vi "CapsLockEvent.vi"(0 "Input String":string, 7 "stop":bool) -> ()   [LabVIEW 2020]
doc: "This VI is done to implement keyboard , panel based filtering event to change the common functionality\nand configure it as per our requirement"
panel:
  # "Enter the input string to test the caps lock event \nand the front panel close is mapped to close and \ntermination of the program"
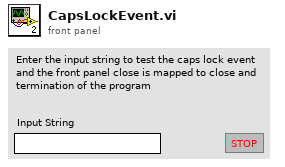
[diagram p1: front panel]
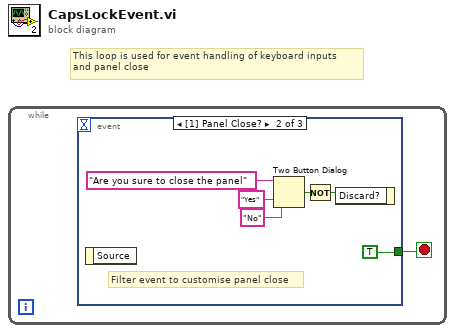
[diagram p0: block diagram]
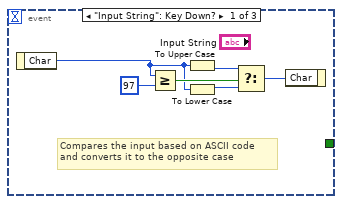
[diagram p2: hidden frame]
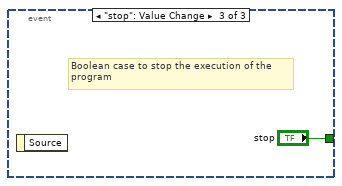
[diagram p3: hidden frame]
diagram:
  # "This loop is used for event handling of keyboard inputs\nand panel close"
  n1 = while {
    stop <- w1 stop-if-true
    n2 = event shown="[1] Panel Close?" {
      selector: _ -> [_ _ _]
      dyn-events: _ -> [_ _ _]
      timeout: _ -> [_ _ _]
      tunnel: [_ TRUE ("y") "stop"] -> w1
      event "Input String": Key Down? {
        # "Compares the input based on ASCII code\nand converts it to the opposite case"
        n3 = event-data() -> ("Char"=w5:i16)  [unwired: 1 in]
        n4 = Greater Or Equal?(x=w5, y=i16 97) -> (x >= y?=w7:bool)
        n5 = To Upper Case(1:w5) -> (0:w3:i16)
        n6 = To Lower Case(string=w5) -> (all lower case string=w4:i16)
        n7 = Select(t=w3, s=w7, f=w4) -> (s? t:f=w2:i16)
        n8 = event-data("Char"=w2) -> ()  [unwired: 1 in, 1 out]
      }
      event Panel Close? {
        # "Filter event to customise panel close"
        n9 = event-data() -> ()  [unwired: 1 in, 1 out]
        n10 = Two Button Dialog(message="Are you sure to close the panel", 1:"No" ("F button name (\"Cancel\")"), 2:"Yes" ("T button name (\"OK\")")) -> (T button?=w10:bool)
        n11 = Not(x=w10) -> (.not. x?=w9:bool)
        n12 = event-data("Discard?"=w9) -> ()  [unwired: 1 in, 1 out]
      }
      event "stop": Value Change {
        # "Boolean case to stop the execution of the \nprogram"
        n13 = event-data() -> ()  [unwired: 1 in, 1 out]
      }
    }
  }
